vi "Read Path Configuration.vi"(8 "error in (no error)":errorcluster, 9 "Default If Not Found":path=path "", 10 "Name":string, 11 "database-configuration in":refnum<class "configuration-database.lvclass">) -> (0 "error out":errorcluster, 1 "Not Found?":bool, 2 "Value":path, 3 "database-configuration out":refnum<class "configuration-database.lvclass">)   [LabVIEW 2020, in "configuration-database.lvlib" / "configuration-database.lvclass"]
uses:
  configuration-database.lvclass
  configuration-database.lvclass/configuration-database.ctl
  be5cd2d0-8ae8-4a6f-b291-74a1993646db.vi
  <vilib>/Utility/error.llb/Error Cluster From Error Code.vi
  IConfigDBQueries/IConfigurationDatabaseQueries.lvclass
  externals/database-interface/IDatabase/IDatabase/IDatabase.lvclass
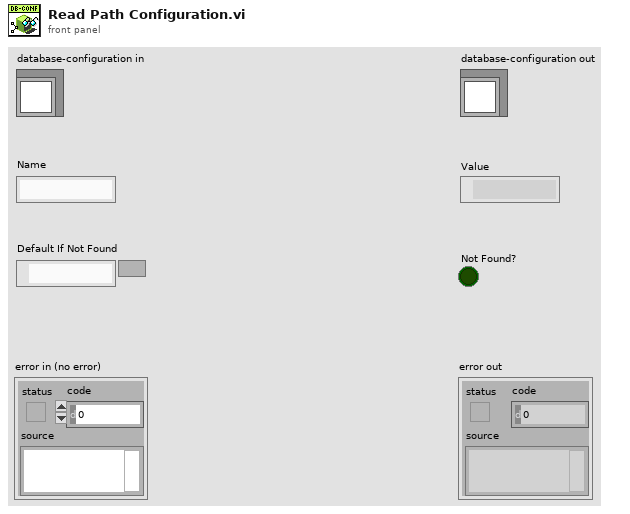
[diagram p1: front panel]
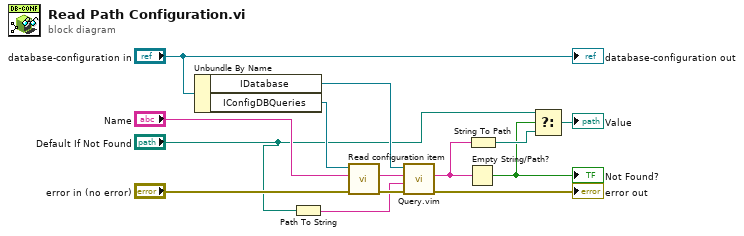
[diagram p0: block diagram]
diagram:
  n1 = Unbundle By Name("database-configuration in") -> ("IDatabase"=w13:refnum<class "IDatabase.lvclass">, "IConfigDBQueries"=w14:refnum<class "IConfigurationDatabaseQueries.lvclass">)
  n2 = Path To String(path="Default If Not Found") -> (string=w1:string)
  n3 = call-dynamic "Read configuration item.vi"("error in (no error)"="error in (no error)", "configuration item"="Name", "IConfigDBQueries in"=w14) -> ("error out"=w12:errorcluster, "result"=w11:string)  [unwired: 7 in]
  n4 = call "Query.vim"("error in (no error)"=w12, "Type and Default"=w1, "Query string"=w11, "IDatabase in"=w13) -> ("error out"=→"error out":errorcluster, "Result"=w7:string)  [unwired: 5 in, 1 out]
  n5 = Empty String/Path?(string/path=w7) -> (empty?=w4:bool)
  "Not Found?" <- w4
  n6 = String To Path(string=w7) -> (path=w10:path)
  n7 = Select(t="Default If Not Found", s=w4, f=w10) -> (s? t:f=→"Value":path)
  "database-configuration out" <- "database-configuration in"
